vi "Write to RT.vi"(8 "error in (no error)":errorcluster, 9 "data words":u16[](array[numeric]), 10 "number of words":u16, 11 "rt transfer handle":u64) -> (0 "error out":errorcluster)   [LabVIEW 2023, in "Ballard MIL-STD-1553 Engine Support.lvlib" / "Implementation.lvlib" / "Tx Execution Unit.lvclass"]
uses:
  Tx Execution Unit.lvclass
  <instrlib>/BTI1553Lib/BTI1553LV.lvlib
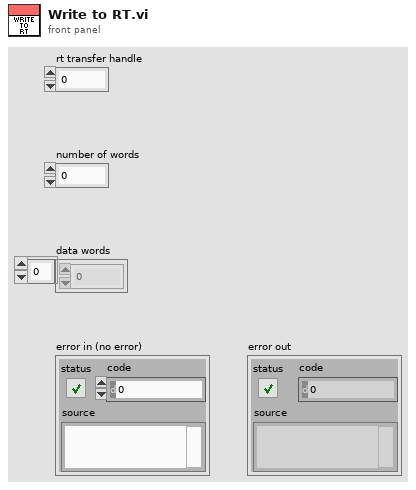
[diagram p1: front panel]
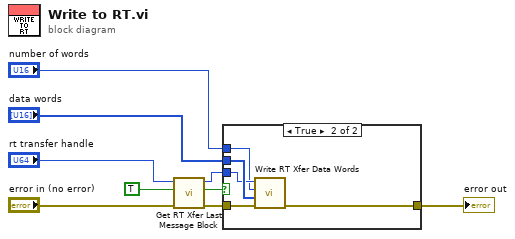
[diagram p0: block diagram]
diagram:
  n1 = call <instrlib>:"Get RT Xfer Last Message Block.vi"("error in (no error)"="error in (no error)", "clear hit?"=TRUE, "rt transfer handle in"="rt transfer handle") -> ("error out"=w5:errorcluster, "was hit?"=w1:bool, "rt transfer handle out"=w2:u64)  [unwired: 5 in, 1 out]
  n2 = case shown="True" w1 {
    tunnel: w5 -> [w10 w15]
    tunnel: "data words" -> [_ w14]
    tunnel: w2 -> [_ w13]
    tunnel: "number of words" -> [_ w12]
    tunnel: [w10 w11] -> w7
    frame False {
    }
    frame True {
      n3 = call <instrlib>:"Write RT Xfer Data Words.vi"("error in (no error)"=w15, "data words"=w14, "data word count in"=w12, "rt transfer handle in"=w13) -> ("error out"=w11:errorcluster)  [unwired: 5 in, 2 out]
    }
  }
  "error out" <- w7
